vi "socket_char_data.vi"() -> ()   [LabVIEW 2019]
panel:
  out "data out":string
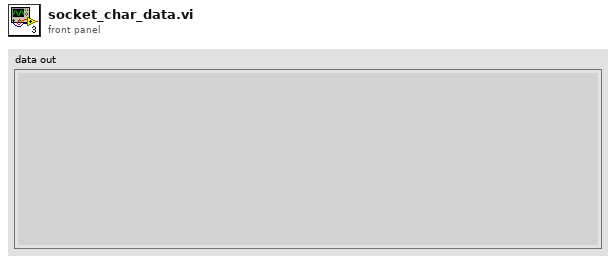
[diagram p1: front panel]
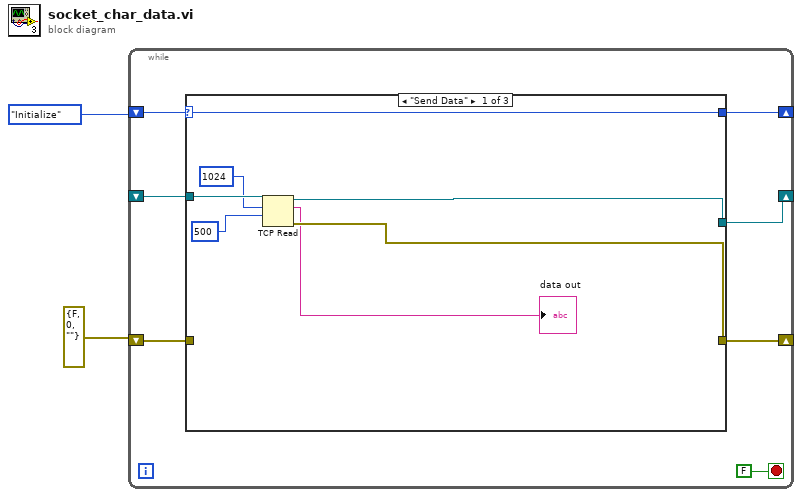
[diagram p0: block diagram]
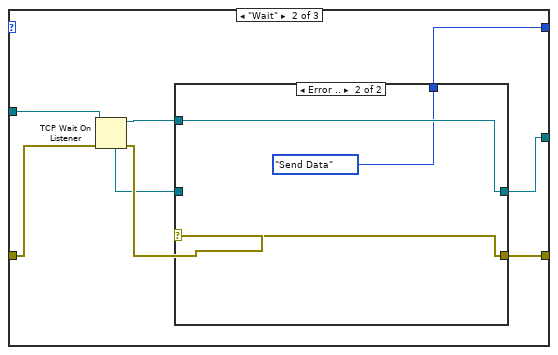
[diagram p2: hidden frame]
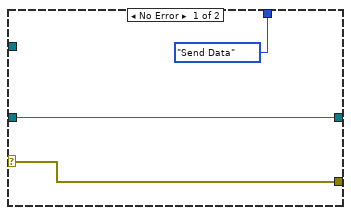
[diagram p3: hidden frame]
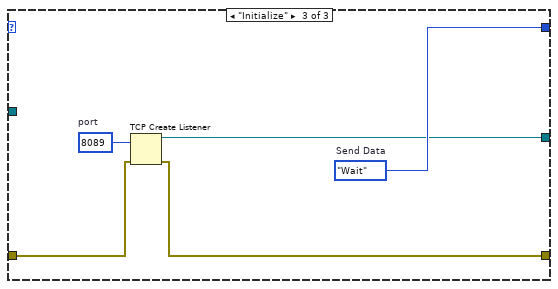
[diagram p4: hidden frame]
diagram:
  n1 = while {
    shift-right: [w8] -> _
    shift-left: enum16{"Initialize", "Send Data", "Wait"}."Initialize" -> [w9]
    shift-right: [w7] -> _
    shift-left: _ -> [w6]
    shift-right: [w3] -> _
    shift-left: errorcluster {"status"=FALSE, "code"=0, "source"=""} ("error in (no error)") -> [w4]
    stop <- FALSE stop-if-true
    n2 = case shown="\"Send Data\"" w9 {
      selector: w9 -> [w12 _ _]
      tunnel: [w12 w21 w34] -> w8
      tunnel: [w13 w19 w33] -> w7
      tunnel: w6 -> [w16 w24 _]
      tunnel: w4 -> [_ w23 w32]
      tunnel: [w11 w17 w31] -> w3
      frame "Send Data" {
        n3 = TCP Read(connection ID=w16, bytes to read=1024, 9:500 ("timeout ms (25000)")) -> (connection ID out=w13:refnum<k5>, data out=→"data out":string, error out=w11:errorcluster)  [unwired: 1 in, 1 out]
      }
      frame "Wait" {
        n4 = TCP Wait On Listener(8:w23, 11:w24) -> (0:w22:errorcluster, 3:w18:refnum<k5>, 4:w20:refnum<k5>)  [unwired: 4 out]
        n5 = case shown="Error .." w22 {
          selector: w22 -> [w25 w28]
          tunnel: [enum16{"Initialize", "Send Data", "Wait"}."Send Data" enum16{"Initialize", "Send Data", "Wait"}."Send Data"] -> w21
          tunnel: w20 -> [w26 _]
          tunnel: [w26 w30] -> w19
          tunnel: w18 -> [_ w30]
          tunnel: [w25 w28] -> w17
          frame No Error {
          }
          frame Error {
          }
        }
      }
      frame "Initialize" {
        w34 = enum16{"Initialize", "Send Data", "Wait"}."Wait"  # Send Data
        w35 = u16 8089  # port
        n6 = TCP Create Listener(8:w32, 10:w35) -> (0:w31:errorcluster, 3:w33:refnum<k5>)  [unwired: 4 out]
      }
    }
  }
